vi "Post Launch Init.vi"(8 "error in":errorcluster, 11 "Manual UI in":refnum<class "Manual UI.lvclass">) -> (0 "error out":errorcluster, 3 "Manual UI out":refnum<class "Manual UI.lvclass">, 4 "Events":T1, 6 "Self Enqueuer":refnum<class "Message Enqueuer.lvclass">)   [LabVIEW 2019, in "Manual UI.lvlib" / "Manual UI.lvclass"]
uses:
  Project/Manual UI.lvclass
  C:/Users/Public/Documents/Development/builds/Engine/Engine.lvlibp/Project/Engine.lvclass
  builds/Engine/Panel.lvlibp/Panel Helper/Panel Events.ctl
  builds/Engine/Panel.lvlibp/Panel Helper/Events.ctl
  builds/Engine/Engine.lvlibp/Custom Controls/System Events.ctl
  builds/Engine/Engine.lvlibp/Custom Controls/System Status.ctl
  builds/Engine/Engine.lvlibp/Custom Controls/Manual Events.ctl
  builds/Engine/Engine.lvlibp/Custom Controls/UUT_Events.ctl
  builds/Engine/Actor Framework.lvlibp/1abvi3w/vi.lib/ActorFramework/Message Enqueuer/Message Enqueuer.lvclass
  builds/Engine/Engine.lvlibp/Accessors/Read Events.vi
  builds/Engine/Panel Manager.lvlibp/Panel Actor/Panel Actor.lvclass
  C:/Users/Public/Documents/Development/builds/Engine/Panel Manager.lvlibp/Panel Actor/Panel Actor.lvclass
  builds/Engine/Panel.lvlibp/Panel Helper/Panel Helper.lvclass
  builds/Engine/Engine.lvlibp/Project/Engine.lvclass
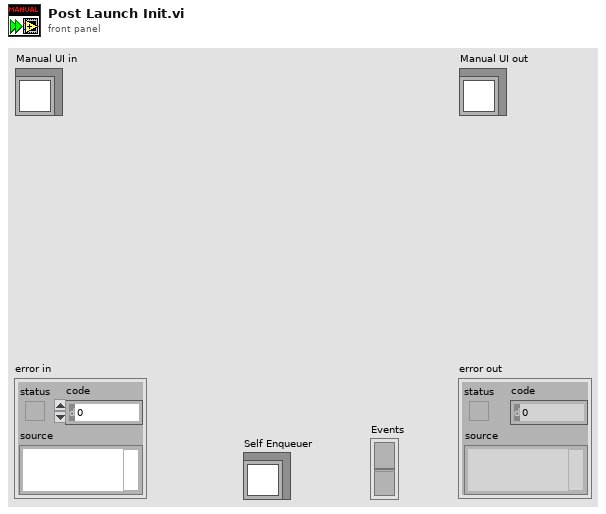
[diagram p1: front panel]
types:
  T1 = cluster{"Pnl Actor":refnum<event-registration>, "Event Registration Refnum":refnum<event-registration>}
  T2 = typedef "Engine.lvlibp/Engine.lvclass/Engine Events.ctl" = cluster{"System Event":T3, "Manual":T4, "UUT":T5, "Interface Events":T6}
  T3 = typedef "Engine.lvlibp/Engine.lvclass/System Events.ctl" = cluster{"Fault Event":refnum<user-event>, "SystemStatus Event":refnum<user-event>, "Automation":refnum<user-event>}
  T4 = typedef "Engine.lvlibp/Engine.lvclass/Manual Events.ctl" = cluster{"QuickStart Event":refnum<user-event>, "SafeBTE Event":refnum<user-event>, "TogglePower Event":refnum<user-event>, "Change Instrument Event":refnum<user-event>, "Toggle Launch Event":refnum<user-event>, "UUTSupply":refnum<user-event>}
  T5 = typedef "Engine.lvlibp/Engine.lvclass/UUT_Events.ctl" = cluster{"UUT_Name":refnum<user-event>, "Test_Name":refnum<user-event>, "Test_Operator":refnum<user-event>, "Test_Witness":refnum<user-event>, "Pedigree_Event":refnum<user-event>}
  T6 = typedef "Engine.lvlibp/Engine.lvclass/Interface Events.ctl" = cluster{"Interface_Command":refnum<user-event>, "Telemetry_Descriptor":refnum<user-event>, "AsynchTLM_Descriptor":refnum<user-event>}
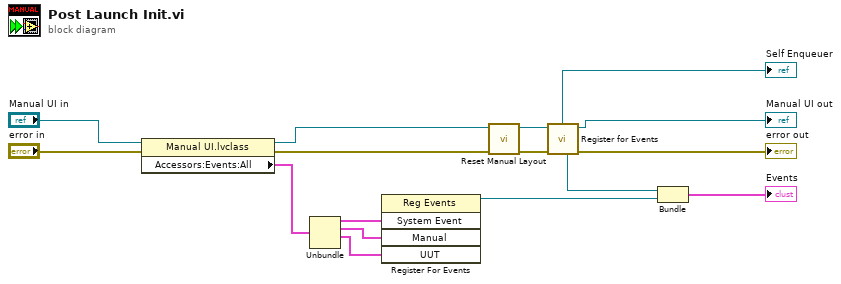
[diagram p0: block diagram]
diagram:
  n1 = property class="Manual UI.lvclass"(reference="Manual UI in", error in="error in") -> (reference out=w10:refnum<class "Manual UI.lvclass">, error out=w9:errorcluster, "Accessors:Events:All"=w8:T2)
  n2 = Unbundle(w8) -> ("System Event"=w5:T3, "Manual"=w4:T4, "UUT"=w3:T5)  [unwired: 1 out]
  n3 = register-events(w5, w4, w3) -> (reference out=w6:refnum<event-registration>)  [unwired: 2 in, 1 out]
  n4 = call-dynamic "Reset Manual Layout.vi"("error in"=w9, "Manual UI in"=w10) -> ("error out"=w15:errorcluster, "Manual UI out"=w16:refnum<class "Manual UI.lvclass">)  [unwired: 8 in]
  n5 = call "Register for Events.vi"("Error In"=w15, "Panel Actor in"=w16) -> ("Error Out"=→"error out":errorcluster, "Panel Actor out"=→"Manual UI out":refnum<class "Manual UI.lvclass">, "Pnl Actor"=w7:refnum<event-registration>, "Self Enqueuer"=→"Self Enqueuer":refnum<class "Message Enqueuer.lvclass">)  [unwired: 6 in]
  n6 = Bundle("Pnl Actor"=w7, "Event Registration Refnum"=w6) -> (→"Events":T1)  [unwired: 1 in]
